vi "myRIO_BRig_Host_v0,33.vi"() -> ()   [LabVIEW 2014]
panel:
  out "error_LoadPrevSettings":errorcluster caption="error out"
  in  "LoadPrevSettings":bool
  out "graph_ai1":dbl(graph)
  out "graph_ai0":dbl(graph)
  in  "dataIn_maxTrialsDisplayed":i32 caption="Number of Trials Displayed\n( 0 = all trials )"
  out "error_TCP":errorcluster
  in  "stop":bool
  in  "colorIn_timeout":u32(colorbox)=7468543 caption="Choice Timeout"
  in  "colorIn_wrong/cue":u32(colorbox)=16728618 caption="Wrong Choice or\nLicked During Cue"
  in  "colorIn_reward":u32(colorbox)=5898088 caption="Reward"
  in  "colorIn_unknown":u32(colorbox)=16449331 caption="Unknown Trial Status"
  out "dataOut_plot":cluster{i32[], i32[]}[](graph)
  out "iTrial":i32
  out "iBlock":i32
  # "Exp Stats"
  # "Current Block Stats"
  # "Trials 2 Reward\n\nBad Trials\nPost Reward"
  # "Left Spout    Right Spout"
  # "Run Time\n\n   minutes    seconds"
  # "Average Block Stats"
  # "Trials 2 Reward\n\nBad Trials\nPost Reward"
  # "Left Spout    Right Spout"
  # "If you get ERROR 5 related to opening a file, press CONTINUE"
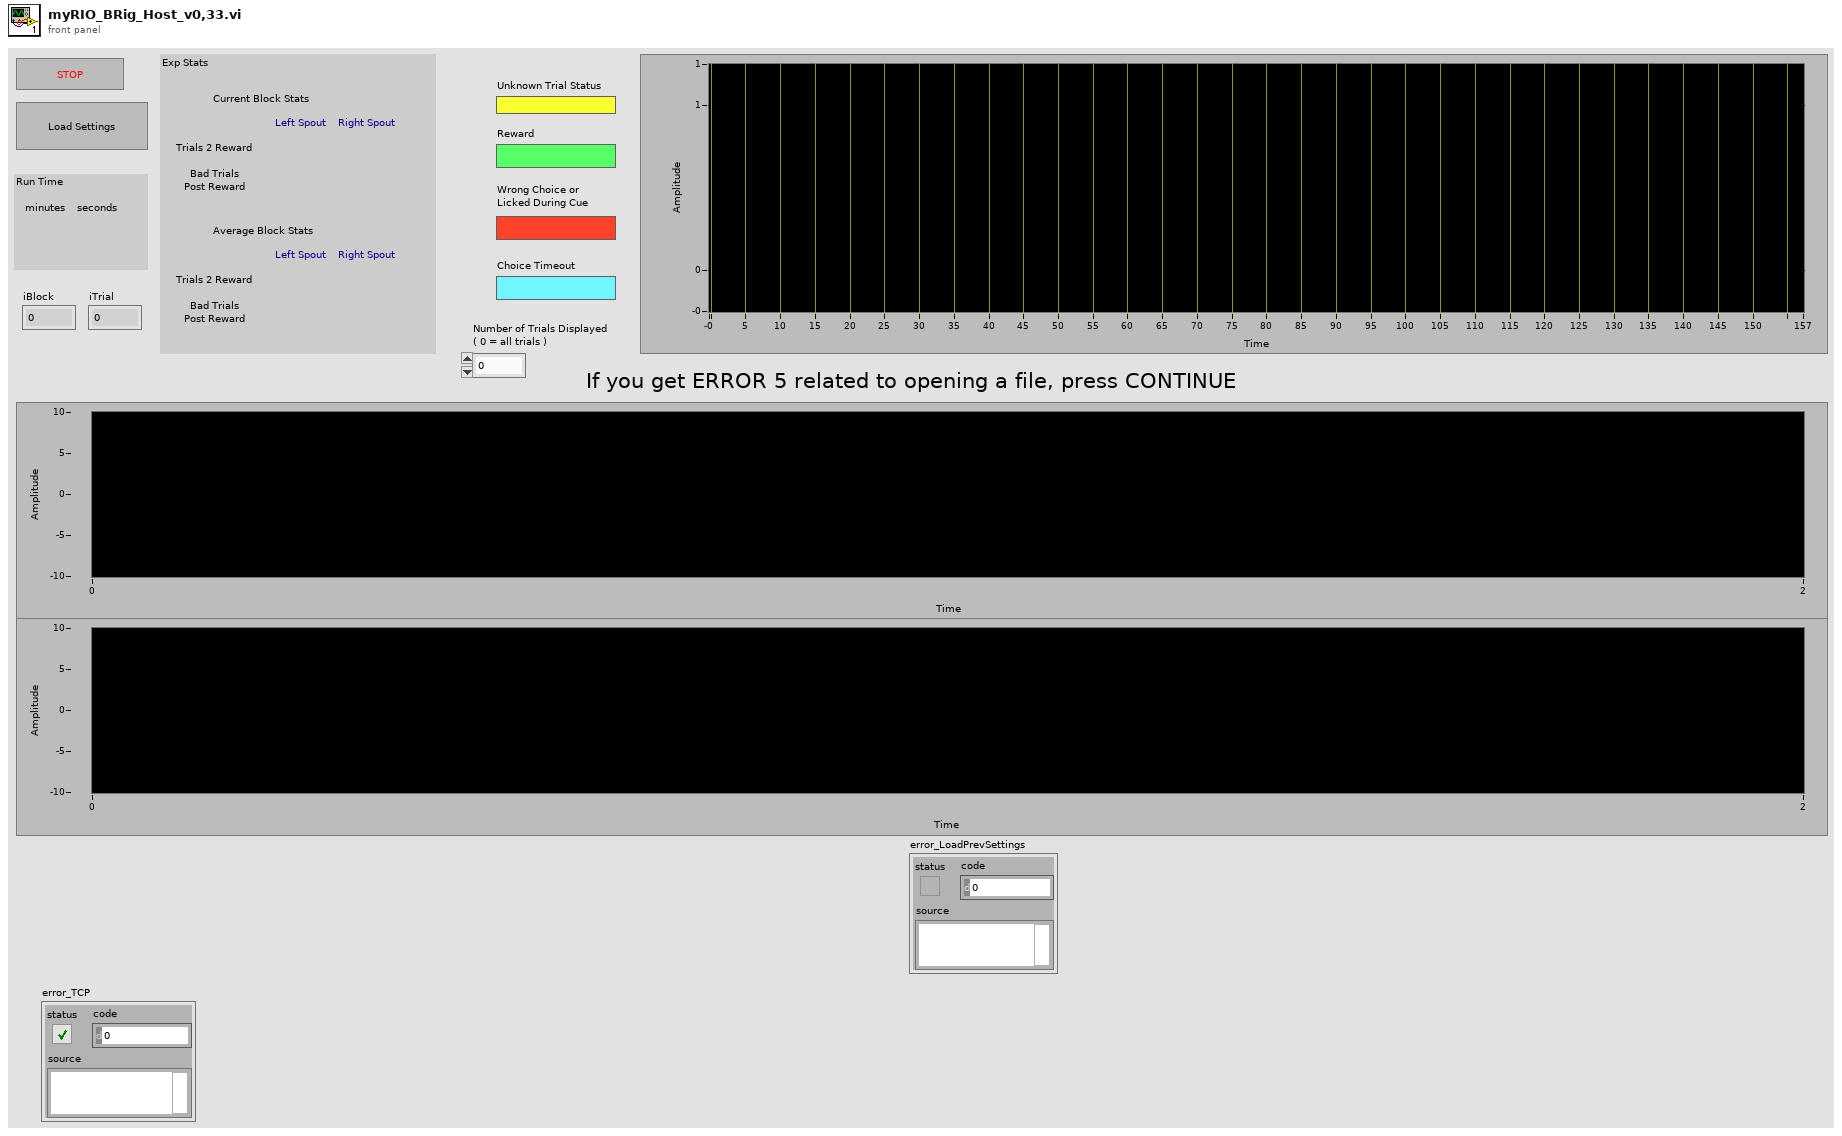
[diagram p1: front panel]
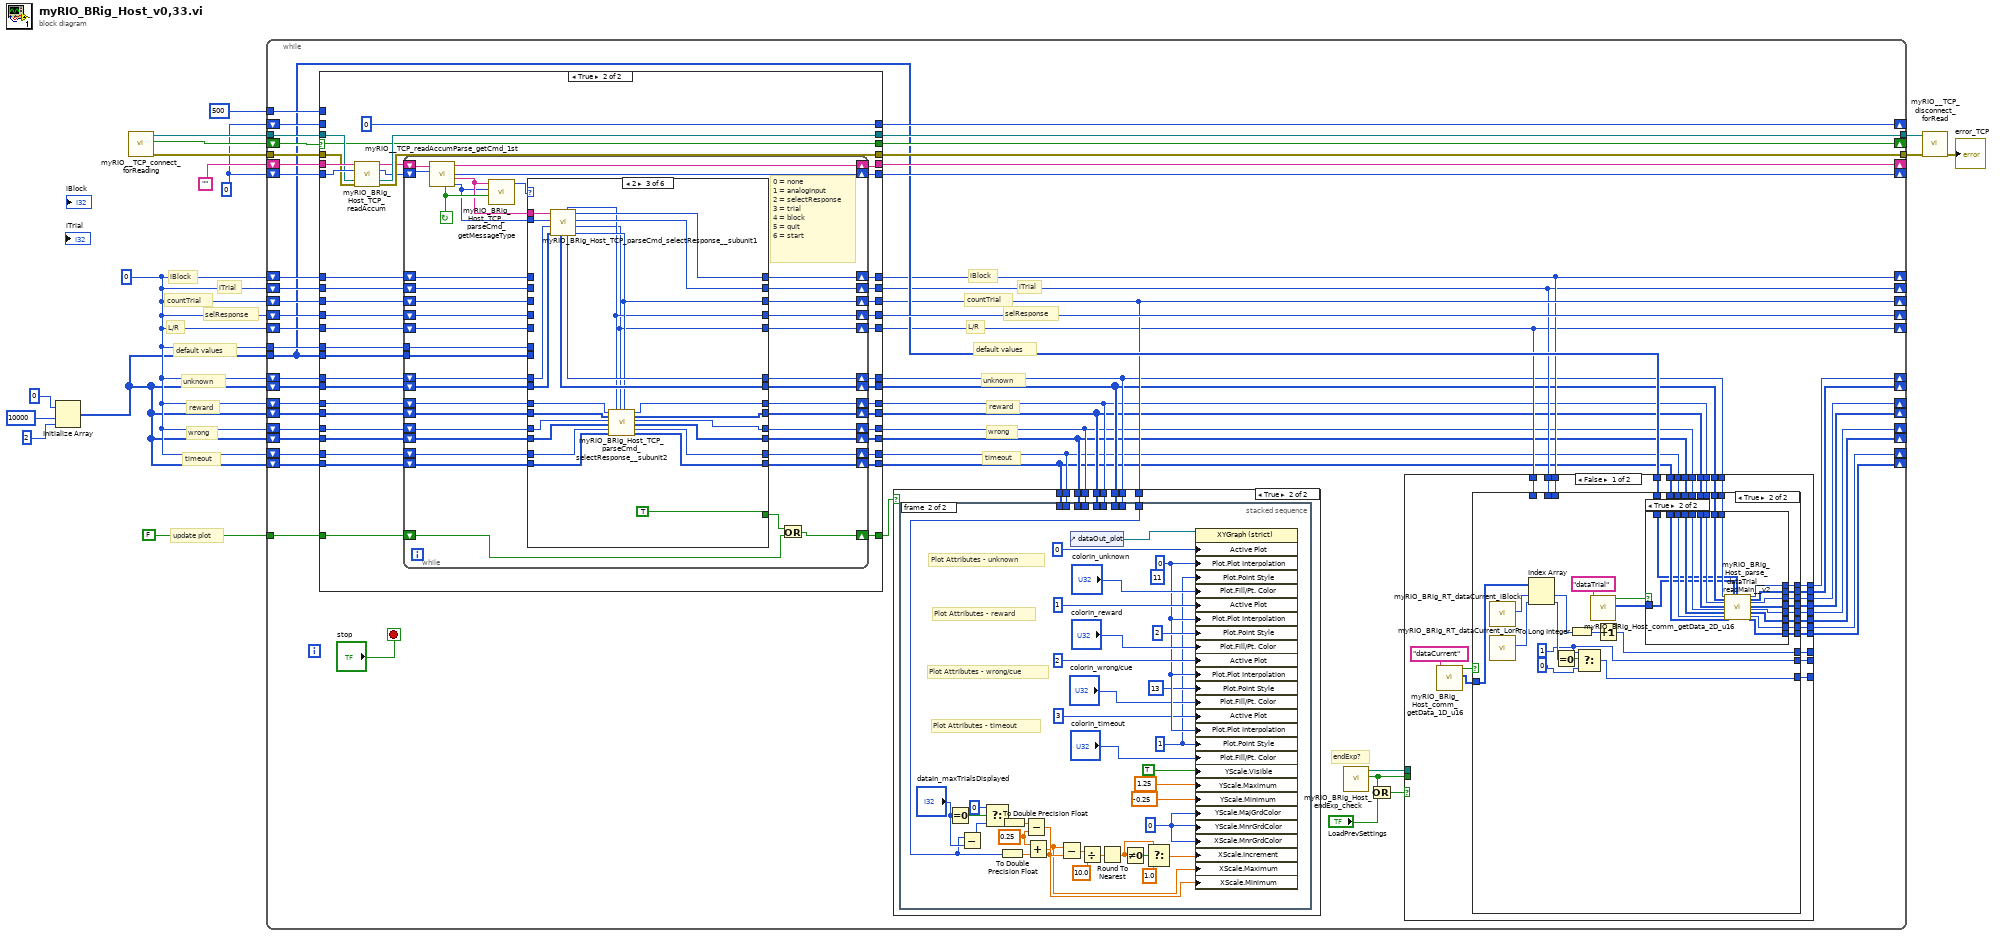
[diagram p0: block diagram]
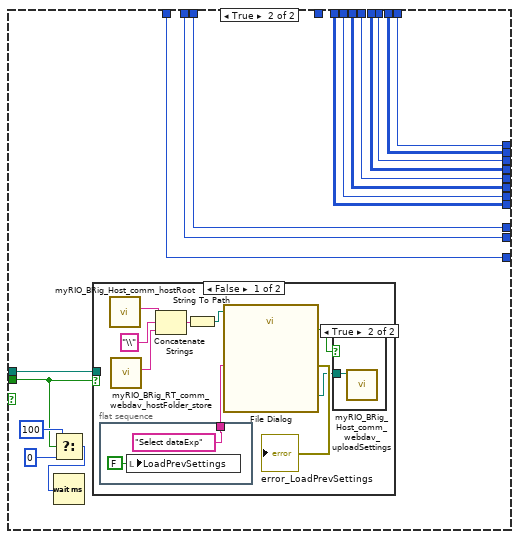
[diagram p4: hidden frame]
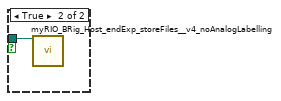
[diagram p6: hidden frame]
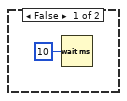
[diagram p7: hidden frame]
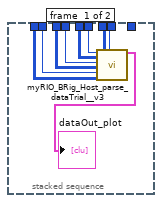
[diagram p8: hidden frame]
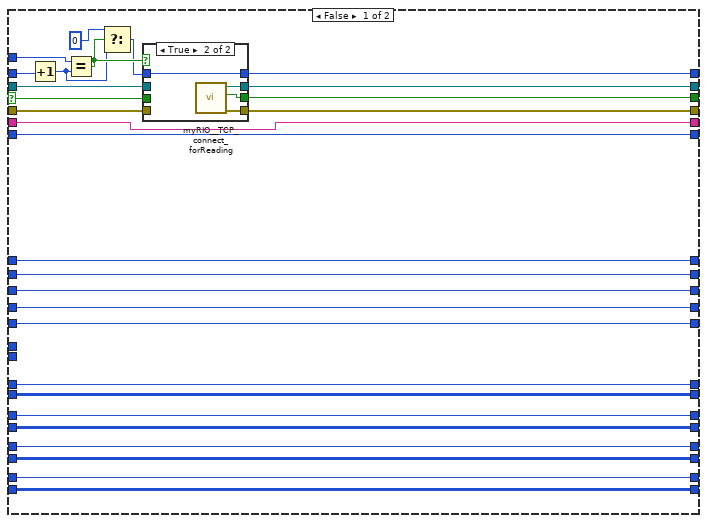
[diagram p9: hidden frame]
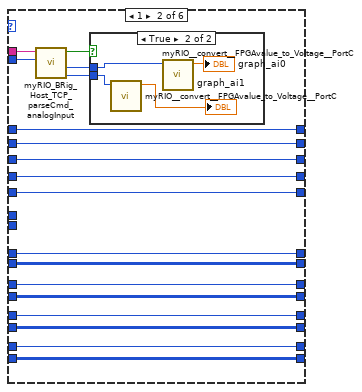
[diagram p12: hidden frame]
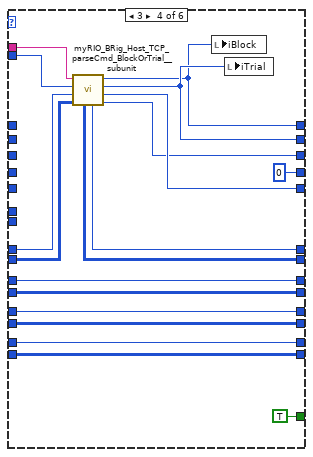
[diagram p14: hidden frame]
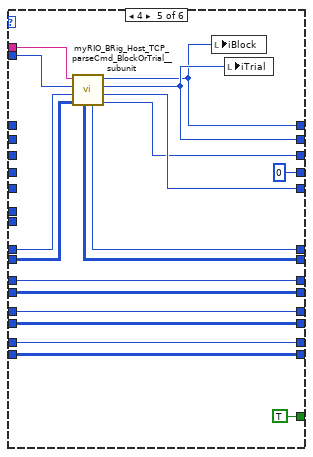
[diagram p15: hidden frame]
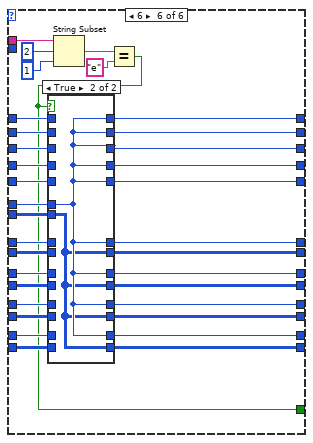
[diagram p16: hidden frame]
diagram:
  w2 = 0
  w11 = 0
  # "default values"
  # "update plot"
  # "timeout"
  # "wrong"
  # "reward"
  # "unknown"
  # "L/R"
  # "selResponse"
  # "countTrial"
  # "iBlock"
  # "iTrial"
  n1 = Initialize Array(0 ("element"), 10000 ("dimension size"), 2 ("dimension size")) -> (w1:i32[][])
  n2 = call "myRIO__TCP_connect_forReading.vi"() -> ("output_error"=w13:errorcluster, "output_connected"=w14:bool, "output_hTCP"=w15:refnum<k5>)  [unwired: 9 in]
  n3 = while {
    tunnel: w15 -> [w70]
    tunnel: w13 -> [w68]
    shift-right: [w61] -> _
    shift-left: w11 -> [w66]
    shift-right: [w62] -> _
    shift-left: "" -> [w67]
    shift-right: [w63] -> _
    shift-left: w14 -> [w69]
    shift-right: [w64] -> _
    shift-left: w11 -> [w71]
    tunnel: 500 ("y") -> [w65]
    shift-right: [w34] -> _
    shift-left: w2 -> [w60]
    shift-right: [w33] -> _
    shift-left: w2 -> [w59]
    shift-right: [w35] -> _
    shift-left: w2 -> [w58]
    shift-right: [w46] -> _
    shift-left: w2 -> [w57]
    shift-right: [w32] -> _
    shift-left: w2 -> [w56]
    shift-right: [w23] -> _
    shift-left: w2 -> [w55]
    shift-right: [w22] -> _
    shift-left: w1 -> [w54]
    shift-right: [w21] -> _
    shift-left: w2 -> [w53]
    shift-right: [w20] -> _
    shift-left: w1 -> [w52]
    shift-right: [w19] -> _
    shift-left: w2 -> [w51]
    shift-right: [w18] -> _
    shift-left: w1 -> [w50]
    shift-right: [w17] -> _
    shift-left: w2 -> [w49]
    shift-right: [w16] -> _
    shift-left: w1 -> [w48]
    tunnel: [w44] -> w5
    tunnel: [w43] -> w4
    tunnel: FALSE -> [w47]
    tunnel: w2 -> [w41]
    tunnel: w1 -> [w36]
    stop <- "stop" stop-if-true
    # "default values"
    # "timeout"
    # "wrong"
    # "reward"
    # "unknown"
    # "L/R"
    # "selResponse"
    # "countTrial"
    # "iBlock"
    # "iTrial"
    # "endExp?"
    n4 = case shown="True" w69 {
      selector: w69 -> [w271 w320]
      tunnel: w67 -> [w265 w326]
      tunnel: w66 -> [w266 w325]
      tunnel: [w265 w316] -> w62
      tunnel: [w266 w315] -> w61
      tunnel: w70 -> [w272 w324]
      tunnel: [w275 w323] -> w44
      tunnel: w68 -> [w270 w322]
      tunnel: [w274 w321] -> w43
      tunnel: [w273 w320] -> w63
      tunnel: w71 -> [w276 _]
      tunnel: [w264 0] -> w64
      tunnel: w65 -> [w263 _]
      tunnel: w60 -> [w262 w314]
      tunnel: w59 -> [w261 w313]
      tunnel: w58 -> [w260 w312]
      tunnel: w57 -> [w259 w311]
      tunnel: w56 -> [w258 w310]
      tunnel: w55 -> [w257 w309]
      tunnel: w54 -> [w256 w308]
      tunnel: w53 -> [w255 w307]
      tunnel: w52 -> [w254 w306]
      tunnel: w51 -> [w253 w305]
      tunnel: w50 -> [w252 w304]
      tunnel: w49 -> [w251 w303]
      tunnel: w48 -> [w250 w302]
      tunnel: w47 -> [_ w301]
      tunnel: [_ w300] -> w45
      tunnel: [w262 w299] -> w34
      tunnel: [w261 w298] -> w33
      tunnel: [w260 w297] -> w35
      tunnel: [w259 w296] -> w46
      tunnel: [w258 w295] -> w32
      tunnel: [w257 w294] -> w31
      tunnel: [w256 w293] -> w30
      tunnel: [w255 w292] -> w29
      tunnel: [w254 w291] -> w28
      tunnel: [w253 w290] -> w27
      tunnel: [w252 w289] -> w26
      tunnel: [w251 w288] -> w25
      tunnel: [w250 w287] -> w24
      tunnel: w41 -> [_ w286]
      tunnel: w36 -> [_ w285]
      frame False {
        n5 = Increment(x=w276) -> (x+1=w249:i32)
        n6 = Equal?(x=w263, y=w249) -> (x = y?=w269:bool)
        n7 = Select(t=0, s=w269, f=w249) -> (s? t:f=w267:i32)
        n8 = case shown="True" w269 {
          tunnel: w267 -> [w277 w281]
          tunnel: [w280 w284] -> w275
          tunnel: [w278 w283] -> w274
          tunnel: [w279 w282] -> w273
          tunnel: w272 -> [w280 _]
          tunnel: w271 -> [w279 _]
          tunnel: w270 -> [w278 _]
          tunnel: [w277 w281] -> w264
          frame False {
          }
          frame True {
            n9 = call "myRIO__TCP_connect_forReading.vi"() -> ("output_error"=w283:errorcluster, "output_connected"=w282:bool, "output_hTCP"=w284:refnum<k5>)  [unwired: 9 in]
          }
        }
      }
      frame True {
        n10 = call "myRIO_BRig_Host_TCP_readAccum.vi"("input_strAccum"=w326, "input_count"=w325, "input_handle_TCP"=w324, "input_error"=w322) -> ("output_strAccum"=w318:string, "output_count"=w317:i32, "output_handle_TCP"=w323:refnum<k5>, "output_error"=w321:errorcluster)  [unwired: 8 in]
        n11 = while {
          shift-right: [w363] -> w316
          shift-left: w318 -> [w365]
          shift-right: [w362] -> w315
          shift-left: w317 -> [w364]
          shift-right: [w354] -> w299
          shift-left: w314 -> [w357]
          shift-right: [w353] -> w298
          shift-left: w313 -> [w356]
          shift-right: [w352] -> w297
          shift-left: w312 -> [w355]
          shift-right: [w350] -> w296
          shift-left: w311 -> [w351]
          shift-right: [w348] -> w295
          shift-left: w310 -> [w349]
          shift-right: [w346] -> w294
          shift-left: w309 -> [w347]
          shift-right: [w344] -> w293
          shift-left: w308 -> [w345]
          shift-right: [w337] -> w292
          shift-left: w307 -> [w343]
          shift-right: [w336] -> w291
          shift-left: w306 -> [w342]
          shift-right: [w335] -> w290
          shift-left: w305 -> [w341]
          shift-right: [w334] -> w289
          shift-left: w304 -> [w340]
          shift-right: [w332] -> w287
          shift-left: w302 -> [w338]
          shift-right: [w333] -> w288
          shift-left: w303 -> [w339]
          shift-right: [w330] -> w300
          shift-left: w301 -> [w327]
          tunnel: w286 -> [w329]
          tunnel: w285 -> [w328]
          stop <- w361 continue-if-true
          # "0 = none\n1 = analogInput\n2 = selectResponse\n3 = trial\n4 = block\n5 = quit\n6 = start"
          n12 = call "myRIO__TCP_readAccumParse_getCmd_1st.vi"("input_count"=w364, "input_strAccum"=w365) -> ("output_countCmd"=w359:i32, "output_strCmd"=w360:string, "output_count"=w362:i32, "output_strAccum"=w363:string, "output_haveCmd"=w361:bool)  [unwired: 5 in]
          n13 = call "myRIO_BRig_Host_TCP_parseCmd_getMessageType.vi"("input_haveCmd"=w361, "input_countCmd"=w359, "input_strCmd"=w360) -> ("output_messageType"=w358:u8)  [unwired: 8 in]
          n14 = case shown="2" w358 {
            tunnel: w360 -> [_ w383 w424 w441 w459 w494]
            tunnel: w359 -> [_ w382 w423 w440 w458 _]
            tunnel: w357 -> [w378 w396 _ _ _ w489]
            tunnel: w356 -> [w377 w395 _ _ _ w487]
            tunnel: w355 -> [w376 w394 _ _ _ w486]
            tunnel: [w378 w396 w418 w426 w444 w488] -> w354
            tunnel: [w377 w395 w417 w427 w445 w483] -> w353
            tunnel: [w376 w394 w416 w434 w452 w482] -> w352
            tunnel: w351 -> [w375 w393 _ _ _ w485]
            tunnel: [w375 w393 w415 0 ("output_iTrial_num") 0 ("output_iTrial_num") w481] -> w350
            tunnel: w349 -> [w374 w392 _ _ _ w484]
            tunnel: [w374 w392 w414 w435 w453 w480] -> w348
            tunnel: w347 -> [w373 w391 w422 w439 w457 w479]
            tunnel: [w373 w391 w420 w437 w455 w471] -> w346
            tunnel: w345 -> [w372 w390 w421 w438 w456 w478]
            tunnel: [w372 w390 w419 w436 w454 w470] -> w344
            tunnel: w343 -> [w371 w389 w413 w433 w451 w477]
            tunnel: w342 -> [w370 w388 w412 w432 w450 w476]
            tunnel: w341 -> [w369 w387 w411 w431 w449 w475]
            tunnel: w340 -> [w368 w386 w410 w430 w448 w474]
            tunnel: w339 -> [w367 w385 w409 w429 w447 w473]
            tunnel: w338 -> [w366 w384 w408 w428 w446 w472]
            tunnel: [w371 w389 w407 w433 w451 w469] -> w337
            tunnel: [w370 w388 w406 w432 w450 w468] -> w336
            tunnel: [w369 w387 w405 w431 w449 w467] -> w335
            tunnel: [w368 w386 w404 w430 w448 w466] -> w334
            tunnel: [w367 w385 w403 w429 w447 w465] -> w333
            tunnel: [w366 w384 w402 w428 w446 w464] -> w332
            tunnel: [_ _ TRUE TRUE TRUE w461] -> w331
            tunnel: w329 -> [_ _ _ _ _ w463]
            tunnel: w328 -> [_ _ _ _ _ w462]
            frame 0, Default {
            }
            frame 1 {
              n15 = call "myRIO_BRig_Host_TCP_parseCmd_analogInput.vi"("input_countCmd"=w382, "input_strCmd"=w383) -> ("output_ai1"=w379:i32, "output_ai0"=w380:i32, "output_haveAnalogInput"=w381:bool)  [unwired: 7 in]
              n16 = case shown="True" w381 {
                tunnel: w380 -> [_ w400]
                tunnel: w379 -> [_ w398]
                frame False {
                }
                frame True {
                  n17 = call "myRIO__convert__FPGAvalue_to_Voltage__PortC.vi"("input_FPGAvalue_PortC"=w398) -> ("output_voltage"=→"graph_ai1":dbl)  [unwired: 10 in]
                  n18 = call "myRIO__convert__FPGAvalue_to_Voltage__PortC.vi"("input_FPGAvalue_PortC"=w400) -> ("output_voltage"=→"graph_ai0":dbl)  [unwired: 10 in]
                }
              }
            }
            frame 2 {
              n19 = call "myRIO_BRig_Host_TCP_parseCmd_selectResponse__subunit1.vi"("input_arrayUnknown"=w421, "input_idxUnknown"=w422, "input_countCmd"=w423, "input_strCmd"=w424) -> ("output_countTrial"=w416:i32, "output_L/R"=w414:i32, "output_iTrial"=w417:i32, "output_iBlock"=w418:i32, "output_idxUnknown"=w420:i32, "output_response"=w415:i32, "output_arrayUnknown"=w419:i32[][])  [unwired: 1 in]
              n20 = call "myRIO_BRig_Host_TCP_parseCmd_selectResponse__subunit2.vi"("input_idxReward"=w413, "input_arrayReward"=w412, "input_idxWrong"=w411, "input_arrayWrong"=w410, "input_idxTimeout"=w409, "input_arrayTimeout"=w408, "input_response"=w415, "input_L/R"=w414, "input_countTrial"=w416) -> ("output_idxReward"=w407:i32, "output_arrayReward"=w406:i32[][], "output_idxWrong"=w405:i32, "output_arrayWrong"=w404:i32[][], "output_idxTimeout"=w403:i32, "output_arrayTimeout"=w402:i32[][])  [unwired: 5 in]
            }
            frame 3 {
              n21 = call "myRIO_BRig_Host_TCP_parseCmd_BlockOrTrial__subunit.vi"("input_arrayUnknown"=w438, "input_idxUnknown"=w439, "input_countCmd"=w440, "input_strCmd"=w441) -> ("output_countTrial"=w434:i32, "output_L/R"=w435:i32, "output_iTrial"=w427:i32, "output_iBlock"=w426:i32, "output_idxUnknown"=w437:i32, "output_arrayUnknown"=w436:i32[][])  [unwired: 2 in]
              n22 = local write "iBlock"(w426) -> ()
              n23 = local write "iTrial"(w427) -> ()
            }
            frame 4 {
              n24 = call "myRIO_BRig_Host_TCP_parseCmd_BlockOrTrial__subunit.vi"("input_arrayUnknown"=w456, "input_idxUnknown"=w457, "input_countCmd"=w458, "input_strCmd"=w459) -> ("output_countTrial"=w452:i32, "output_L/R"=w453:i32, "output_iTrial"=w445:i32, "output_iBlock"=w444:i32, "output_idxUnknown"=w455:i32, "output_arrayUnknown"=w454:i32[][])  [unwired: 2 in]
              n25 = local write "iBlock"(w444) -> ()
              n26 = local write "iTrial"(w445) -> ()
            }
            frame 6 {
              n27 = String Subset(string=w494, offset (0)=2, length (rest)=1 ("length (rest)")) -> (substring=w491:string)
              n28 = Equal?(x=w491, y="e") -> (x = y?=w461:bool)
              n29 = case shown="True" w461 {
                tunnel: w489 -> [w507 _]
                tunnel: [w507 w509] -> w488
                tunnel: w487 -> [w506 _]
                tunnel: w486 -> [w505 _]
                tunnel: w485 -> [w504 _]
                tunnel: w484 -> [w503 _]
                tunnel: [w506 w509] -> w483
                tunnel: [w505 w509] -> w482
                tunnel: [w504 w509] -> w481
                tunnel: [w503 w509] -> w480
                tunnel: w479 -> [w502 _]
                tunnel: w478 -> [w501 _]
                tunnel: w477 -> [w500 _]
                tunnel: w476 -> [w499 _]
                tunnel: w475 -> [w498 _]
                tunnel: w474 -> [w497 _]
                tunnel: w473 -> [w496 _]
                tunnel: w472 -> [w495 _]
                tunnel: [w502 w509] -> w471
                tunnel: [w501 w508] -> w470
                tunnel: [w500 w509] -> w469
                tunnel: [w499 w508] -> w468
                tunnel: [w498 w509] -> w467
                tunnel: [w497 w508] -> w466
                tunnel: [w496 w509] -> w465
                tunnel: [w495 w508] -> w464
                tunnel: w463 -> [_ w509]
                tunnel: w462 -> [_ w508]
                frame False {
                }
                frame True {
                }
              }
            }
          }
          n30 = Or(x=w331, y=w327) -> (x .or. y?=w330:bool)
        }
      }
    }
    n31 = case shown="True" w45 {
      tunnel: w24 -> [_ w204]
      tunnel: w25 -> [_ w203]
      tunnel: w26 -> [_ w202]
      tunnel: w27 -> [_ w201]
      tunnel: w28 -> [_ w200]
      tunnel: w29 -> [_ w199]
      tunnel: w30 -> [_ w198]
      tunnel: w31 -> [_ w197]
      tunnel: w35 -> [_ w196]
      frame False {
        n32 = Wait (ms)(milliseconds to wait=u32 10) -> ()  [unwired: 1 out]
      }
      frame True {
        n33 = stacked-sequence {
          tunnel: w204 -> [w213 _]
          tunnel: w203 -> [w212 _]
          tunnel: w202 -> [w211 _]
          tunnel: w201 -> [w210 _]
          tunnel: w200 -> [w209 _]
          tunnel: w199 -> [w208 _]
          tunnel: w198 -> [w207 _]
          tunnel: w197 -> [w206 _]
          tunnel: w196 -> [_ w222]
          frame #0 {
            n34 = call "myRIO_BRig_Host_parse_dataTrial__v3.vi"("input_idxReward"=w208, "input_arrayReward"=w209, "input_idxWrong"=w210, "input_arrayWrong"=w211, "input_idxTimeout"=w212, "input_arrayTimeout"=w213, "input_arrayUnknown"=w207, "input_idxUnknown"=w206) -> ("output_plotData"=→"dataOut_plot":cluster{i32[], i32[]}[])  [unwired: 11 in]
          }
          frame #1 {
            w218 = u32 0 ("Y Scale.Grid Colors:Major Color")
            w226 = 0.25 ("y")
            w215 = u8 1 ("Plot.Point Style")
            (unwired) u8 11 ("Plot.Point Style")
            w242 = u8 0 ("Plot.Plot Interpolation")
            # "Plot Attributes - timeout"
            # "Plot Attributes - wrong/cue"
            # "Plot Attributes - reward"
            # "Plot Attributes - unknown"
            n35 = Equal To 0?(x="dataIn_maxTrialsDisplayed") -> (x = 0?=w223:bool)
            n36 = Subtract(x=w222, y="dataIn_maxTrialsDisplayed") -> (x-y=w224:i32)
            n37 = Select(t=0, s=w223, f=w224) -> (s? t:f=w229:i32)
            n38 = To Double Precision Float(number=w222) -> (double precision float=w227:dbl)
            n39 = To Double Precision Float(number=w229) -> (double precision float=w228:dbl)
            n40 = Subtract(x=w228, y=w226) -> (x-y=w216:dbl)
            n41 = Add(x=w226, y=w227) -> (x+y=w214:dbl)
            n42 = Subtract(x=w214, y=w216) -> (x-y=w230:dbl)
            n43 = control-ref of="dataOut_plot"() -> (w237:refnum<vi>)
            n44 = Divide(x=w230, y=10.0) -> (x/y=w232:dbl)
            n45 = Round To Nearest(number=w232) -> (nearest integer value=w234:dbl)
            n46 = Not Equal To 0?(x=w234) -> (x != 0?=w233:bool)
            n47 = Select(t=w234, s=w233, f=1.0) -> (s? t:f=w217:dbl)
            n48 = property on="Property Node" class="XYGraph (strict)"(reference=w237, "Active Plot"=u32 0, "Plot.Plot Interpolation"=w242, "Plot.Point Style"=w215, "Plot.Fill/Pt. Color"="colorIn_unknown", "Active Plot"=u32 1, "Plot.Plot Interpolation"=w242, "Plot.Point Style"=u8 2, "Plot.Fill/Pt. Color"="colorIn_reward", "Active Plot"=u32 2, "Plot.Plot Interpolation"=w242, "Plot.Point Style"=u8 13, "Plot.Fill/Pt. Color"="colorIn_wrong/cue", "Active Plot"=u32 3, "Plot.Plot Interpolation"=w242, "Plot.Point Style"=w215, "Plot.Fill/Pt. Color"="colorIn_timeout", "YScale.Visible"=TRUE ("Y Scale.Visible"), "YScale.Maximum"=1.25 ("Y Scale.Range:Maximum"), "YScale.Minimum"=-0.25 ("Y Scale.Range:Minimum"), "YScale.MajGrdColor"=w218, "YScale.MnrGrdColor"=w218, "XScale.MnrGrdColor"=w218, "XScale.Increment"=w217, "XScale.Maximum"=w214, "XScale.Minimum"=w216) -> ()  [unwired: 1 in, 2 out]
          }
        }
      }
    }
    n49 = call "myRIO_BRig_Host_endExp_check.vi"() -> ("output_IendExp"=w38:bool, "output_filePath_expExp"=w37:path)  [unwired: 10 in]
    n50 = Or(x=w38, y="LoadPrevSettings") -> (x .or. y?=w39:bool)
    n51 = case shown="False" w39 {
      tunnel: w38 -> [_ w178]
      tunnel: w37 -> [_ w177]
      tunnel: [w94 w176] -> w23
      tunnel: [w93 w175] -> w22
      tunnel: [w92 w174] -> w21
      tunnel: [w91 w173] -> w20
      tunnel: [w90 w172] -> w19
      tunnel: [w89 w171] -> w18
      tunnel: [w88 w170] -> w17
      tunnel: [w87 w169] -> w16
      tunnel: w31 -> [w86 w176]
      tunnel: w30 -> [w85 w175]
      tunnel: w29 -> [w84 w174]
      tunnel: w28 -> [w83 w173]
      tunnel: w27 -> [w82 w172]
      tunnel: w26 -> [w81 w171]
      tunnel: w25 -> [w80 w170]
      tunnel: w24 -> [w79 w169]
      tunnel: w36 -> [w78 _]
      tunnel: [w77 w166] -> _
      tunnel: [w76 w167] -> _
      tunnel: [w75 w168] -> _
      tunnel: w34 -> [w74 w168]
      tunnel: w33 -> [w73 w167]
      tunnel: w32 -> [w72 w166]
      frame False {
        n52 = call "myRIO_BRig_Host_comm_getData_1D_u16.vi"("input_fileName"="dataCurrent") -> ("output_data_1D"=w95:u16[], "output_I_data"=w96:bool)  [unwired: 9 in]
        n53 = case shown="True" w96 {
          tunnel: w95 -> [_ w139]
          tunnel: [w108 w134] -> w94
          tunnel: [w107 w133] -> w93
          tunnel: [w106 w132] -> w92
          tunnel: [w105 w131] -> w91
          tunnel: [w104 w130] -> w90
          tunnel: [w103 w129] -> w89
          tunnel: [w102 w128] -> w88
          tunnel: [w101 w127] -> w87
          tunnel: w86 -> [w108 w126]
          tunnel: w85 -> [w107 w125]
          tunnel: w84 -> [w106 w124]
          tunnel: w83 -> [w105 w123]
          tunnel: w82 -> [w104 w122]
          tunnel: w81 -> [w103 w121]
          tunnel: w80 -> [w102 w120]
          tunnel: w79 -> [w101 w119]
          tunnel: w78 -> [_ w118]
          tunnel: [w98 w114] -> w77
          tunnel: [w99 w113] -> w76
          tunnel: [w100 w109] -> w75
          tunnel: w74 -> [w100 _]
          tunnel: w73 -> [w99 _]
          tunnel: w72 -> [w98 _]
          frame False {
          }
          frame True {
            w113 = 1
            n54 = call "myRIO_BRig_RT_dataCurrent_iBlock.vi"() -> ("output_iBlock"=w112:i32)  [unwired: 11 in]
            n55 = call "myRIO_BRig_RT_dataCurrent_LorR.vi"() -> ("output_LorR"=w135:i32)  [unwired: 11 in]
            n56 = Index Array(array=w139, index #1=w112, index #2=w135) -> (element #1=w111:u16, element #2=w117:u16)
            n57 = Equal To 0?(x=w117) -> (x = 0?=w116:bool)
            n58 = To Long Integer(number=w111) -> (32bit integer=w110:i32)
            n59 = Select(t=w113, s=w116, f=0) -> (s? t:f=w114:i32)
            n60 = call "myRIO_BRig_Host_comm_getData_2D_u16.vi"("input_fileName"="dataTrial") -> ("output_data_2D"=w136:u16[][], "output_I_data"=w137:bool)  [unwired: 9 in]
            n61 = Increment(x=w110) -> (x+1=w109:i32)
            n62 = case shown="True" w137 {
              tunnel: w136 -> [_ w157]
              tunnel: [w145 w153] -> w132
              tunnel: [w144 w152] -> w131
              tunnel: [w146 w154] -> w133
              tunnel: [w147 w155] -> w134
              tunnel: [w143 w151] -> w130
              tunnel: [w142 w150] -> w129
              tunnel: [w141 w149] -> w128
              tunnel: [w140 w148] -> w127
              tunnel: w118 -> [_ w156]
              tunnel: w126 -> [w147 w165]
              tunnel: w125 -> [w146 w164]
              tunnel: w124 -> [w145 w163]
              tunnel: w123 -> [w144 w162]
              tunnel: w122 -> [w143 w161]
              tunnel: w121 -> [w142 w160]
              tunnel: w120 -> [w141 w159]
              tunnel: w119 -> [w140 w158]
              frame False {
              }
              frame True {
                n63 = call "myRIO_BRig_Host_parse_dataTrial__readMain__v2.vi"("input_idxUnknown"=w165, "input_arrayUnknown"=w164, "input_idxReward"=w163, "input_arrayReward"=w162, "input_idxWrong"=w161, "input_arrayWrong"=w160, "input_idxTimeout"=w159, "input_arrayTimeout"=w158, "arrayIn_dataTrial"=w157, "arrayIn_empty"=w156) -> ("output_idxUnknown"=w155:i32, "output_arrayUnknown"=w154:i32[][], "output_idxReward"=w153:i32, "output_arrayReward"=w152:i32[][], "output_idxWrong"=w151:i32, "output_arrayWrong"=w150:i32[][], "output_idxTimeout"=w149:i32, "output_arrayTimeout"=w148:i32[][])  [unwired: 10 in]
              }
            }
          }
        }
      }
      frame True {
        n64 = Select(t=u32 100 ("milliseconds to wait"), s=w178, f=u32 0 ("milliseconds to wait")) -> (s? t:f=w180:u32)
        n65 = Wait (ms)(milliseconds to wait=w180) -> ()  [unwired: 1 out]
        n66 = case shown="False" w178 {
          tunnel: w177 -> [_ w194]
          frame False {
            n67 = flat-sequence {
              tunnel: ["Select dataExp" ("prompt")] -> w185
              frame #0 {
                n68 = local write "LoadPrevSettings"(FALSE ("LoadPrevSettings")) -> ()
              }
            }
            n69 = call "myRIO_BRig_Host_comm_hostRoot.vi"() -> ("output_hostRoot"=w187:string)  [unwired: 11 in]
            n70 = call "myRIO_BRig_RT_comm_webdav_hostFolder_store.vi"() -> ("output_HostFolder"=w189:string)  [unwired: 11 in]
            n71 = Concatenate Strings(w187, "\\" ("string"), w189) -> (w190:string)
            n72 = String To Path(string=w190) -> (path=w186:path)
            n73 = call "File Dialog"("start path"=w186, "prompt"=w185) -> ("selected path"=w182:path, "exists"=w183:bool, "error out"=→"error_LoadPrevSettings":errorcluster)  [unwired: 10 in, 1 out]
            n74 = case shown="True" w183 {
              tunnel: w182 -> [_ w191]
              frame False {
              }
              frame True {
                n75 = call "myRIO_BRig_Host_comm_webdav_uploadSettings.vi"("input_filePath"=w191) -> ()  [unwired: 11 in]
              }
            }
          }
          frame True {
            n76 = call "myRIO_BRig_Host_endExp_storeFiles__v4_noAnalogLabelling.vi"("input_filePath"=w194) -> ()  [unwired: 15 in]
          }
        }
      }
    }
  }
  n77 = call "myRIO__TCP_disconnect_forRead.vi"("input_error"=w4, "input_hTCP"=w5) -> ("output_error"=→"error_TCP":errorcluster)  [unwired: 9 in]
